vi "capCalc_rad.vi"(7 "[uF/cm²]     default membran capacity":dbl, 8 "capOut Ch4":dbl, 9 "capOut Ch3":dbl, 10 "capOut Ch2":dbl, 11 "capOut Ch1":dbl) -> (0 "Ch4Rad":dbl, 1 "Ch3Rad":dbl, 2 "Ch2Rad":dbl, 3 "Ch1Rad":dbl)   [LabVIEW 2021]
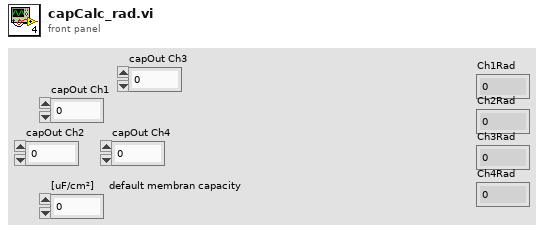
[diagram p1: front panel]
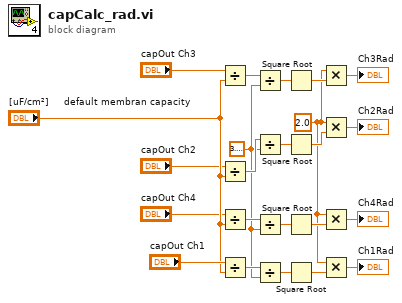
[diagram p0: block diagram]
diagram:
  w2 = 2.0 ("x")
  w1 = 3.141592653589793
  n1 = Divide(x="capOut Ch3", y="[uF/cm²]     default membran capacity") -> (x/y=w13:dbl)
  n2 = Divide(x="capOut Ch2", y="[uF/cm²]     default membran capacity") -> (x/y=w18:dbl)
  n3 = Divide(x="capOut Ch4", y="[uF/cm²]     default membran capacity") -> (x/y=w12:dbl)
  n4 = Divide(x="capOut Ch1", y="[uF/cm²]     default membran capacity") -> (x/y=w20:dbl)
  n5 = Divide(x=w13, y=w1) -> (x/y=w14:dbl)
  n6 = Divide(x=w18, y=w1) -> (x/y=w17:dbl)
  n7 = Divide(x=w12, y=w1) -> (x/y=w11:dbl)
  n8 = Divide(x=w20, y=w1) -> (x/y=w21:dbl)
  n9 = Square Root(x=w14) -> (sqrt(x)=w15:dbl)
  n10 = Square Root(x=w17) -> (sqrt(x)=w16:dbl)
  n11 = Square Root(x=w11) -> (sqrt(x)=w10:dbl)
  n12 = Square Root(x=w21) -> (sqrt(x)=w22:dbl)
  n13 = Multiply(x=w2, y=w15) -> (x*y=→"Ch3Rad":dbl)
  n14 = Multiply(x=w2, y=w16) -> (x*y=→"Ch2Rad":dbl)
  n15 = Multiply(x=w2, y=w10) -> (x*y=→"Ch4Rad":dbl)
  n16 = Multiply(x=w2, y=w22) -> (x*y=→"Ch1Rad":dbl)
